vi "canDataSort.vi"() -> ()   [LabVIEW 2023] (continued)
 00000004    8        00\t00\tFF\tFF\tFF\tFF\tFF\tFF\r\n      2683  0CF102A7   00000004    8        30\t75\tE0\t2E\t80\tFF\tFF\tFD\r\n      2683  0CF101A7   00000004    8        68\t00\t97\tCC\t00\t16\t39\tA0\r\n      2682  1FFFFFFF   00000004    8        00\t20\tFF\tFF\tFF\tFF\tFF\tFF\r\n      2672  1FFFFFFF   00000004    8        00\t00\tFF\tFF\tFF\tFF\tFF\tFF\r\n      2663  0CF102A7   00000004    8        30\t75\tE0\t2E\t80\tFF\tFF\tFD\r\n      2663  0CF101A7   00000004    8        68\t00\t97\tCC\t00\t16\t39\t9F\r\n      2662  1FFFFFFF   00000004    8        00\t00\tFF\tFF\tFF\tFF\tFF\tFF\r\n      2652  1FFFFFFF   00000004    8        00\t00\tFF\tFF\tFF\tFF\tFF\tFF\r\n      2703  0CF101A7   00000004    8        68\t00\t97\tCC\t00\t16\t39\tA1\r\n      2702  1FFFFFFF   00000004    8        00\t00\tFF\tFF\tFF\tFF\tFF\tFF\r\n      2693  18F106A7   00000004    8        00\tF7\tFF\tFF\tFF\tFF\tFF\tA6\r\n      2692  1FFFFFFF   00000004    8        00\t00\tFF\tFF\tFF\tFF\tFF\tFF\r\n      2683  0CF102A7   00000004    8        30\t75\tE0\t2E\t80\tFF\tFF\tFD\r\n      2683  0CF101A7   00000004    8        68\t00\t97\tCC\t00\t16\t39\tA0\r\n      2682  1FFFFFFF   00000004    8        00\t20\tFF\tFF\tFF\tFF\tFF\tFF\r\n      2672  1FFFFFFF   00000004    8        00\t00\tFF\tFF\tFF\tFF\tFF\tFF\r\n      2663  0CF102A7   00000004    8        30\t75\tE0\t2E\t80\tFF\tFF\tFD\r\n      2663  0CF101A7   00000004    8        68\t00\t97\tCC\t00\t16\t39\t9F\r\n      2662  1FFFFFFF   00000004    8        00\t00\tFF\tFF\tFF\tFF\tFF\tFF\r\n      2703  0CF102A7   00000004    8        30\t75\tE0\t2E\t80\tFF\tFF\tFD\r\n      2703  0CF101A7   00000004    8        68\t00\t97\tCC\t00\t16\t39\tA1\r\n      2702  1FFFFFFF   00000004    8        00\t00\tFF\tFF\tFF\tFF\tFF\tFF\r\n      2693  18F106A7   00000004    8        00\tF7\tFF\tFF\tFF\tFF\tFF\tA6\r\n      2692  1FFFFFFF   00000004    8        00\t00\tFF\tFF\tFF\tFF\tFF\tFF\r\n      2683  0CF102A7   00000004    8        30\t75\tE0\t2E\t80\tFF\tFF\tFD\r\n      2683  0CF101A7   00000004    8        68\t00\t97\tCC\t00\t16\t39\tA0\r\n      2682  1FFFFFFF   00000004    8        00\t20\tFF\tFF\tFF\tFF\tFF\tFF\r\n      2672  1FFFFFFF   00000004    8        00\t00\tFF\tFF\tFF\tFF\tFF\tFF\r\n      2663  0CF102A7   00000004    8        30\t75\tE0\t2E\t80\tFF\tFF\tFD\r\n      2663  0CF101A7   00000004    8        68\t00\t97\tCC\t00\t16\t39\t9F\r\n      2712  1FFFFFFF   00000004    8        00\t00\tFF\tFF\tFF\tFF\tFF\tFF\r\n      2703  0CF102A7   00000004    8        30\t75\tE0\t2E\t80\tFF\tFF\tFD\r\n      2703  0CF101A7   00000004    8        68\t00\t97\tCC\t00\t16\t39\tA1\r\n      2702  1FFFFFFF   00000004    8        00\t00\tFF\tFF\tFF\tFF\tFF\tFF\r\n      2693  18F106A7   00000004    8        00\tF7\tFF\tFF\tFF\tFF\tFF\tA6\r\n      2692  1FFFFFFF   00000004    8        00\t00\tFF\tFF\tFF\tFF\tFF\tFF\r\n      2683  0CF102A7   00000004    8        30\t75\tE0\t2E\t80\tFF\tFF\tFD\r\n      2683  0CF101A7   00000004    8        68\t00\t97\tCC\t00\t16\t39\tA0\r\n      2682  1FFFFFFF   00000004    8        00\t20\tFF\tFF\tFF\tFF\tFF\tFF\r\n      2672  1FFFFFFF   00000004    8        00\t00\tFF\tFF\tFF\tFF\tFF\tFF\r\n      2663  0CF102A7   00000004    8        30\t75\tE0\t2E\t80\tFF\tFF\tFD\r\n      2722  1FFFFFFF   00000004    8        00\t00\tFF\tFF\tFF\tFF\tFF\tFF\r\n      2712  1FFFFFFF   00000004    8        00\t00\tFF\tFF\tFF\tFF\tFF\tFF\r\n      2703  0CF102A7   00000004    8        30\t75\tE0\t2E\t80\tFF\tFF\tFD\r\n      2703  0CF101A7   00000004    8        68\t00\t97\tCC\t00\t16\t39\tA1\r\n      2702  1FFFFFFF   00000004    8        00\t00\tFF\tFF\tFF\tFF\tFF\tFF\r\n      2693  18F106A7   00000004    8        00\tF7\tFF\tFF\tFF\tFF\tFF\tA6\r\n      2692  1FFFFFFF   00000004    8        00\t00\tFF\tFF\tFF\tFF\tFF\tFF\r\n      2683  0CF102A7   00000004    8        30\t75\tE0\t2E\t80\tFF\tFF\tFD\r\n      2683  0CF101A7   00000004    8        68\t00\t97\tCC\t00\t16\t39\tA0\r\n      2682  1FFFFFFF   00000004    8        00\t20\tFF\tFF\tFF\tFF\tFF\tFF\r\n      2672  1FFFFFFF   00000004    8        00\t00\tFF\tFF\tFF\tFF\tFF\tFF\r\n      2723  0CF101A7   00000004    8        68\t00\t97\tCC\t00\t16\t39\tA2\r\n      2722  1FFFFFFF   00000004    8        00\t00\tFF\tFF\tFF\tFF\tFF\tFF\r\n      2712  1FFFFFFF   00000004    8        00\t00\tFF\tFF\tFF\tFF\tFF\tFF\r\n      2703  0CF102A7   00000004    8        30\t75\tE0\t2E\t80\tFF\tFF\tFD\r\n      2703  0CF101A7   00000004    8        68\t00\t97\tCC\t00\t16\t39\tA1\r\n      2702  1FFFFFFF   00000004    8        00\t00\tFF\tFF\tFF\tFF\tFF\tFF\r\n      2693  18F106A7   00000004    8        00\tF7\tFF\tFF\tFF\tFF\tFF\tA6\r\n      2692  1FFFFFFF   00000004    8        00\t00\tFF\tFF\tFF\tFF\tFF\tFF\r\n      2683  0CF102A7   00000004    8        30\t75\tE0\t2E\t80\tFF\tFF\tFD\r\n      2683  0CF101A7   00000004    8        68\t00\t97\tCC\t00\t16\t39\tA0\r\n      2682  1FFFFFFF   00000004    8        00\t20\tFF\tFF\tFF\tFF\tFF\tFF\r\n      2723  0CF102A7   00000004    8        30\t75\tE0\t2E\t80\tFF\tFF\tFD\r\n      2723  0CF101A7   00000004    8        68\t00\t97\tCC\t00\t16\t39\tA2\r\n      2722  1FFFFFFF   00000004    8        00\t00\tFF\tFF\tFF\tFF\tFF\tFF\r\n      2712  1FFFFFFF   00000004    8        00\t00\tFF\tFF\tFF\tFF\tFF\tFF\r\n      2703  0CF102A7   00000004    8        30\t75\tE0\t2E\t80\tFF\tFF\tFD\r\n      2703  0CF101A7   00000004    8        68\t00\t97\tCC\t00\t16\t39\tA1\r\n      2702  1FFFFFFF   00000004    8        00\t00\tFF\tFF\tFF\tFF\tFF\tFF\r\n      2693  18F106A7   00000004    8        00\tF7\tFF\tFF\tFF\tFF\tFF\tA6\r\n      2692  1FFFFFFF   00000004    8        00\t00\tFF\tFF\tFF\tFF\tFF\tFF\r\n      2683  0CF102A7   00000004    8        30\t75\tE0\t2E\t80\tFF\tFF\tFD\r\n      2683  0CF101A7   00000004    8        68\t00\t97\tCC\t00\t16\t39\tA0\r\n      2732  1FFFFFFF   00000004    8        00\t00\tFF\tFF\tFF\tFF\tFF\tFF\r\n      2723  0CF102A7   00000004    8        30\t75\tE0\t2E\t80\tFF\tFF\tFD\r\n      2723  0CF101A7   00000004    8        68\t00\t97\tCC\t00\t16\t39\tA2\r\n      2722  1FFFFFFF   00000004    8        00\t00\tFF\tFF\tFF\tFF\tFF\tFF\r\n      2712  1FFFFFFF   00000004    8        00\t00\tFF\tFF\tFF\tFF\tFF\tFF\r\n      2703  0CF102A7   00000004    8        30\t75\tE0\t2E\t80\tFF\tFF\tFD\r\n      2703  0CF101A7   00000004    8        68\t00\t97\tCC\t00\t16\t39\tA1\r\n      2702  1FFFFFFF   00000004    8        00\t00\tFF\tFF\tFF\tFF\tFF\tFF\r\n      2693  18F106A7   00000004    8        00\tF7\tFF\tFF\tFF\tFF\tFF\tA6\r\n      2692  1FFFFFFF   00000004    8        00\t00\tFF\tFF\tFF\tFF\tFF\tFF\r\n      2683  0CF102A7   00000004    8        30\t75\tE0\t2E\t80\tFF\tFF\tFD\r\n      2741  18F11FF0   00000004    8        FF\t3F\t90\t68\t88\t1B\t10\t3C\r\n      2732  1FFFFFFF   00000004    8        00\t00\tFF\tFF\tFF\tFF\tFF\tFF\r\n      2723  0CF102A7   00000004    8        30\t75\tE0\t2E\t80\tFF\tFF\tFD\r\n      2723  0CF101A7   00000004    8        68\t00\t97\tCC\t00\t16\t39\tA2\r\n      2722  1FFFFFFF   00000004    8        00\t00\tFF\tFF\tFF\tFF\tFF\tFF\r\n      2712  1FFFFFFF   00000004    8        00\t00\tFF\tFF\tFF\tFF\tFF\tFF\r\n      2703  0CF102A7   00000004    8        30\t75\tE0\t2E\t80\tFF\tFF\tFD\r\n      2703  0CF101A7   00000004    8        68\t00\t97\tCC\t00\t16\t39\tA1\r\n      2702  1FFFFFFF   00000004    8        00\t00\tFF\tFF\tFF\tFF\tFF\tFF\r\n      2693  18F106A7   00000004    8        00\tF7\tFF\tFF\tFF\tFF\tFF\tA6\r\n      2692  1FFFFFFF   00000004    8        00\t00\tFF\tFF\tFF\tFF\tFF\tFF\r\n      2742  18F120F0   00000004    8        2B\t75\t60\tB1\tB0\t01\tFF\tFF\r\n      2741  18F11FF0   00000004    8        FF\t3F\t90\t68\t88\t1B\t10\t3C\r\n      2732  1FFFFFFF   00000004    8        00\t00\tFF\tFF\tFF\tFF\tFF\tFF\r\n      2723  0CF102A7   00000004    8        30\t75\tE0\t2E\t80\tFF\tFF\tFD\r\n      2723  0CF101A7   00000004    8        68\t00\t97\tCC\t00\t16\t39\tA2\r\n      2722  1FFFFFFF   00000004    8        00\t00\tFF\tFF\tFF\tFF\tFF\tFF\r\n      2712  1FFFFFFF   00000004    8        00\t00\tFF\tFF\tFF\tFF\tFF\tFF\r\n      2703  0CF102A7   00000004    8        30\t75\tE0\t2E\t80\tFF\tFF\tFD\r\n      2703  0CF101A7   00000004    8        68\t00\t97\tCC\t00\t16\t39\tA1\r\n      2702  1FFFFFFF   00000004    8        00\t00\tFF\tFF\tFF\tFF\tFF\tFF\r\n      2693  18F106A7   00000004    8        00\tF7\tFF\tFF\tFF\tFF\tFF\tA6\r\n      2743  0CF101A7   00000004    8        68\t00\t97\tCC\t00\t16\t39\tA3\r\n      2742  18F120F0   00000004    8        2B\t75\t60\tB1\tB0\t01\tFF\tFF\r\n      2741  18F11FF0   00000004    8        FF\t3F\t90\t68\t88\t1B\t10\t3C\r\n      2732  1FFFFFFF   00000004    8        00\t00\tFF\tFF\tFF\tFF\tFF\tFF\r\n      2723  0CF102A7   00000004    8        30\t75\tE0\t2E\t80\tFF\tFF\tFD\r\n      2723  0CF101A7   00000004    8        68\t00\t97\tCC\t00\t16\t39\tA2\r\n      2722  1FFFFFFF   00000004    8        00\t00\tFF\tFF\tFF\tFF\tFF\tFF\r\n      2712  1FFFFFFF   00000004    8        00\t00\tFF\tFF\tFF\tFF\tFF\tFF\r\n      2703  0CF102A7   00000004    8        30\t75\tE0\t2E\t80\tFF\tFF\tFD\r\n      2703  0CF101A7   00000004    8        68\t00\t97\tCC\t00\t16\t39\tA1\r\n      2702  1FFFFFFF   00000004    8        00\t00\tFF\tFF\tFF\tFF\tFF\tFF\r\n      2743  0C3C4D4A   00000004    8        BE\tFF\tFF\t7F\t18\tFF\tFF\t53\r\n      2743  0CF101A7   00000004    8        68\t00\t97\tCC\t00\t16\t39\tA3\r\n      2742  18F120F0   00000004    8        2B\t75\t60\tB1\tB0\t01\tFF\tFF\r\n      2741  18F11FF0   00000004    8        FF\t3F\t90\t68\t88\t1B\t10\t3C\r\n      2732  1FFFFFFF   00000004    8        00\t00\tFF\tFF\tFF\tFF\tFF\tFF\r\n      2723  0CF102A7   00000004    8        30\t75\tE0\t2E\t80\tFF\tFF\tFD\r\n      2723  0CF101A7   00000004    8        68\t00\t97\tCC\t00\t16\t39\tA2\r\n      2722  1FFFFFFF   00000004    8        00\t00\tFF\tFF\tFF\tFF\tFF\tFF\r\n      2712  1FFFFFFF   00000004    8        00\t00\tFF\tFF\tFF\tFF\tFF\tFF\r\n      2703  0CF102A7   00000004    8        30\t75\tE0\t2E\t80\tFF\tFF\tFD\r\n      2703  0CF101A7   00000004    8        68\t00\t97\tCC\t00\t16\t39\tA1\r\n      2744  0CF102A7   00000004    8        30\t75\tE0\t2E\t80\tFF\tFF\tFD\r\n      2743  0C3C4D4A   00000004    8        BE\tFF\tFF\t7F\t18\tFF\tFF\t53\r\n      2743  0CF101A7   00000004    8        68\t00\t97\tCC\t00\t16\t39\tA3\r\n      2742  18F120F0   00000004    8        2B\t75\t60\tB1\tB0\t01\tFF\tFF\r\n      2741  18F11FF0   00000004    8        FF\t3F\t90\t68\t88\t1B\t10\t3C\r\n      2732  1FFFFFFF   00000004    8        00\t00\tFF\tFF\tFF\tFF\tFF\tFF\r\n      2723  0CF102A7   00000004    8        30\t75\tE0\t2E\t80\tFF\tFF\tFD\r\n      2723  0CF101A7   00000004    8        68\t00\t97\tCC\t00\t16\t39\tA2\r\n      2722  1FFFFFFF   00000004    8        00\t00\tFF\tFF\tFF\tFF\tFF\tFF\r\n      2712  1FFFFFFF   00000004    8        00\t00\tFF\tFF\tFF\tFF\tFF\tFF\r\n      2703  0CF102A7   00000004    8        30\t75\tE0\t2E\t80\tFF\tFF\tFD\r\n      2744  0CF103A7   00000004    8        17\t1F\t08\t60\tB1\t1F\t08\t53\r\n      2744  0CF102A7   00000004    8        30\t75\tE0\t2E\t80\tFF\tFF\tFD\r\n      2743  0C3C4D4A   00000004    8        BE\tFF\tFF\t7F\t18\tFF\tFF\t53\r\n      2743  0CF101A7   00000004    8        68\t00\t97\tCC\t00\t16\t39\tA3\r\n      2742  18F120F0   00000004    8        2B\t75\t60\tB1\tB0\t01\tFF\tFF\r\n      2741  18F11FF0   00000004    8        FF\t3F\t90\t68\t88\t1B\t10\t3C\r\n      2732  1FFFFFFF   00000004    8        00\t00\tFF\tFF\tFF\tFF\tFF\tFF\r\n      2723  0CF102A7   00000004    8        30\t75\tE0\t2E\t80\tFF\tFF\tFD\r\n      2723  0CF101A7   00000004    8        68\t00\t97\tCC\t00\t16\t39\tA2\r\n      2722  1FFFFFFF   00000004    8        00\t00\tFF\tFF\tFF\tFF\tFF\tFF\r\n      2712  1FFFFFFF   00000004    8        00\t00\tFF\tFF\tFF\tFF\tFF\tFF\r\n      2745  0CF104A7   00000004    8        F0\t60\t22\tFC\tFF\tFF\tFF\t53\r\n      2744  0CF103A7   00000004    8        17\t1F\t08\t60\tB1\t1F\t08\t53\r\n      2744  0CF102A7   00000004    8        30\t75\tE0\t2E\t80\tFF\tFF\tFD\r\n      2743  0C3C4D4A   00000004    8        BE\tFF\tFF\t7F\t18\tFF\tFF\t53\r\n      2743  0CF101A7   00000004    8        68\t00\t97\tCC\t00\t16\t39\tA3\r\n      2742  18F120F0   00000004    8        2B\t75\t60\tB1\tB0\t01\tFF\tFF\r\n      2741  18F11FF0   00000004    8        FF\t3F\t90\t68\t88\t1B\t10\t3C\r\n      2732  1FFFFFFF   00000004    8        00\t00\tFF\tFF\tFF\tFF\tFF\tFF\r\n      2723  0CF102A7   00000004    8        30\t75\tE0\t2E\t80\tFF\tFF\tFD\r\n      2723  0CF101A7   00000004    8        68\t00\t97\tCC\t00\t16\t39\tA2\r\n      2722  1FFFFFFF   00000004    8        00\t00\tFF\tFF\tFF\tFF\tFF\tFF\r\n      2745  18F106A7   00000004    8        00\tF7\tFF\tFF\tFF\tFF\tFF\tA7\r\n      2745  0CF104A7   00000004    8        F0\t60\t22\tFC\tFF\tFF\tFF\t53\r\n      2744  0CF103A7   00000004    8        17\t1F\t08\t60\tB1\t1F\t08\t53\r\n      2744  0CF102A7   00000004    8        30\t75\tE0\t2E\t80\tFF\tFF\tFD\r\n      2743  0C3C4D4A   00000004    8        BE\tFF\tFF\t7F\t18\tFF\tFF\t53\r\n      2743  0CF101A7   00000004    8        68\t00\t97\tCC\t00\t16\t39\tA3\r\n      2742  18F120F0   00000004    8        2B\t75\t60\tB1\tB0\t01\tFF\tFF\r\n      2741  18F11FF0   00000004    8        FF\t3F\t90\t68\t88\t1B\t10\t3C\r\n      2732  1FFFFFFF   00000004    8        00\t00\tFF\tFF\tFF\tFF\tFF\tFF\r\n      2723  0CF102A7   00000004    8        30\t75\tE0\t2E\t80\tFF\tFF\tFD\r\n      2723  0CF101A7   00000004    8        68\t00\t97\tCC\t00\t16\t39\tA2\r\n      2746  18F121F0   00000004    8        09\t19\t00\t00\tFF\tFF\tB0\t01\r\n      2745  18F106A7   00000004    8        00\tF7\tFF\tFF\tFF\tFF\tFF\tA7\r\n      2745  0CF104A7   00000004    8        F0\t60\t22\tFC\tFF\tFF\tFF\t53\r\n      2744  0CF103A7   00000004    8        17\t1F\t08\t60\tB1\t1F\t08\t53\r\n      2744  0CF102A7   00000004    8        30\t75\tE0\t2E\t80\tFF\tFF\tFD\r\n      2743  0C3C4D4A   00000004    8        BE\tFF\tFF\t7F\t18\tFF\tFF\t53\r\n      2743  0CF101A7   00000004    8        68\t00\t97\tCC\t00\t16\t39\tA3\r\n      2742  18F120F0   00000004    8        2B\t75\t60\tB1\tB0\t01\tFF\tFF\r\n      2741  18F11FF0   00000004    8        FF\t3F\t90\t68\t88\t1B\t10\t3C\r\n      2732  1FFFFFFF   00000004    8        00\t00\tFF\tFF\tFF\tFF\tFF\tFF\r\n      2723  0CF102A7   00000004    8        30\t75\tE0\t2E\t80\tFF\tFF\tFD\r\n      2747  1FFFFFFF   00000004    8        00\t00\tFF\tFF\tFF\tFF\tFF\tFF\r\n      2746  18F121F0   00000004    8        09\t19\t00\t00\tFF\tFF\tB0\t01\r\n      2745  18F106A7   00000004    8        00\tF7\tFF\tFF\tFF\tFF\tFF\tA7\r\n      2745  0CF104A7   00000004    8        F0\t60\t22\tFC\tFF\tFF\tFF\t53\r\n      2744  0CF103A7   00000004    8        17\t1F\t08\t60\tB1\t1F\t08\t53\r\n      2744  0CF102A7   00000004    8        30\t75\tE0\t2E\t80\tFF\tFF\tFD\r\n      2743  0C3C4D4A   00000004    8        BE\tFF\tFF\t7F\t18\tFF\tFF\t53\r\n      2743  0CF101A7   00000004    8        68\t00\t97\tCC\t00\t16\t39\tA3\r\n      2742  18F120F0   00000004    8        2B\t75\t60\tB1\tB0\t01\tFF\tFF\r\n      2741  18F11FF0   00000004    8        FF\t3F\t90\t68\t88\t1B\t10\t3C\r\n      2732  1FFFFFFF   00000004    8        00\t00\tFF\tFF\tFF\tFF\tFF\tFF\r\n      2752  1FFFFFFF   00000004    8        00\t00\tFF\tFF\tFF\tFF\tFF\tFF\r\n      2747  1FFFFFFF   00000004    8        00\t00\tFF\tFF\tFF\tFF\tFF\tFF\r\n      2746  18F121F0   00000004    8        09\t19\t00\t00\tFF\tFF\tB0\t01\r\n      2745  18F106A7   00000004    8        00\tF7\tFF\tFF\tFF\tFF\tFF\tA7\r\n      2745  0CF104A7   00000004    8        F0\t60\t22\tFC\tFF\tFF\tFF\t53\r\n      2744  0CF103A7   00000004    8        17\t1F\t08\t60\tB1\t1F\t08\t53\r\n      2744  0CF102A7   00000004    8        30\t75\tE0\t2E\t80\tFF\tFF\tFD\r\n      2743  0C3C4D4A   00000004    8        BE\tFF\tFF\t7F\t18\tFF\tFF\t53\r\n      2743  0CF101A7   00000004    8        68\t00\t97\tCC\t00\t16\t39\tA3\r\n      2742  18F120F0   00000004    8        2B\t75\t60\tB1\tB0\t01\tFF\tFF\r\n      2741  18F11FF0   00000004    8        FF\t3F\t90\t68\t88\t1B\t10\t3C\r\n      2762  1FFFFFFF   00000004    8        00\t00\tFF\tFF\tFF\tFF\tFF\tFF\r\n      2752  1FFFFFFF   00000004    8        00\t00\tFF\tFF\tFF\tFF\tFF\tFF\r\n      2747  1FFFFFFF   00000004    8        00\t00\tFF\tFF\tFF\tFF\tFF\tFF\r\n      2746  18F121F0   00000004    8        09\t19\t00\t00\tFF\tFF\tB0\t01\r\n      2745  18F106A7   00000004    8        00\tF7\tFF\tFF\tFF\tFF\tFF\tA7\r\n      2745  0CF104A7   00000004    8        F0\t60\t22\tFC\tFF\tFF\tFF\t53\r\n      2744  0CF103A7   00000004    8        17\t1F\t08\t60\tB1\t1F\t08\t53\r\n      2744  0CF102A7   00000004    8        30\t75\tE0\t2E\t80\tFF\tFF\tFD\r\n      2743  0C3C4D4A   00000004    8        BE\tFF\tFF\t7F\t18\tFF\tFF\t53\r\n      2743  0CF101A7   00000004    8        68\t00\t97\tCC\t00\t16\t39\tA3\r\n      2742  18F120F0   00000004    8        2B\t75\t60\tB1\tB0\t01\tFF\tFF\r\n      2763  0CF101A7   00000004    8        68\t00\t97\tCC\t00\t16\t39\tA4\r\n      2762  1FFFFFFF   00000004    8        00\t00\tFF\tFF\tFF\tFF\tFF\tFF\r\n      2752  1FFFFFFF   00000004    8        00\t00\tFF\tFF\tFF\tFF\tFF\tFF\r\n      2747  1FFFFFFF   00000004    8        00\t00\tFF\tFF\tFF\tFF\tFF\tFF\r\n      2746  18F121F0   00000004    8        09\t19\t00\t00\tFF\tFF\tB0\t01\r\n      2745  18F106A7   00000004    8        00\tF7\tFF\tFF\tFF\tFF\tFF\tA7\r\n      2745  0CF104A7   00000004    8        F0\t60\t22\tFC\tFF\tFF\tFF\t53\r\n      2744  0CF103A7   00000004    8        17\t1F\t08\t60\tB1\t1F\t08\t53\r\n      2744  0CF102A7   00000004    8        30\t75\tE0\t2E\t80\tFF\tFF\tFD\r\n      2743  0C3C4D4A   00000004    8        BE\tFF\tFF\t7F\t18\tFF\tFF\t53\r\n      2743  0CF101A7   00000004    8        68\t00\t97\tCC\t00\t16\t39\tA3\r\n      2763  0CF102A7   00000004    8        30\t75\tE0\t2E\t80\tFF\tFF\tFD\r\n      2763  0CF101A7   00000004    8        68\t00\t97\tCC\t00\t16\t39\tA4\r\n      2762  1FFFFFFF   00000004    8        00\t00\tFF\tFF\tFF\tFF\tFF\tFF\r\n      2752  1FFFFFFF   00000004    8        00\t00\tFF\tFF\tFF\tFF\tFF\tFF\r\n      2747  1FFFFFFF   00000004    8        00\t00\tFF\tFF\tFF\tFF\tFF\tFF\r\n      2746  18F121F0   00000004    8        09\t19\t00\t00\tFF\tFF\tB0\t01\r\n      2745  18F106A7   00000004    8        00\tF7\tFF\tFF\tFF\tFF\tFF\tA7\r\n      2745  0CF104A7   00000004    8        F0\t60\t22\tFC\tFF\tFF\tFF\t53\r\n      2744  0CF103A7   00000004    8        17\t1F\t08\t60\tB1\t1F\t08\t53\r\n      2744  0CF102A7   00000004    8        30\t75\tE0\t2E\t80\tFF\tFF\tFD\r\n      2743  0C3C4D4A   00000004    8        BE\tFF\tFF\t7F\t18\tFF\tFF\t53\r\n      2772  1FFFFFFF   00000004    8        00\t00\tFF\tFF\tFF\tFF\tFF\tFF\r\n      2763  0CF102A7   00000004    8        30\t75\tE0\t2E\t80\tFF\tFF\tFD\r\n      2763  0CF101A7   00000004    8        68\t00\t97\tCC\t00\t16\t39\tA4\r\n      2762  1FFFFFFF   00000004    8        00\t00\tFF\tFF\tFF\tFF\tFF\tFF\r\n      2752  1FFFFFFF   00000004    8        00\t00\tFF\tFF\tFF\tFF\tFF\tFF\r\n      2747  1FFFFFFF   00000004    8        00\t00\tFF\tFF\tFF\tFF\tFF\tFF\r\n      2746  18F121F0   00000004    8        09\t19\t00\t00\tFF\tFF\tB0\t01\r\n      2745  18F106A7   00000004    8        00\tF7\tFF\tFF\tFF\tFF\tFF\tA7\r\n      2745  0CF104A7   00000004    8        F0\t60\t22\tFC\tFF\tFF\tFF\t53\r\n      2744  0CF103A7   00000004    8        17\t1F\t08\t60\tB1\t1F\t08\t53\r\n      2744  0CF102A7   00000004    8        30\t75\tE0\t2E\t80\tFF\tFF\tFD\r\n      2782  1FFFFFFF   00000004    8        00\t00\tFF\tFF\tFF\tFF\tFF\tFF\r\n      2772  1FFFFFFF   00000004    8        00\t00\tFF\tFF\tFF\tFF\tFF\tFF\r\n      2763  0CF102A7   00000004    8        30\t75\tE0\t2E\t80\tFF\tFF\tFD\r\n      2763  0CF101A7   00000004    8        68\t00\t97\tCC\t00\t16\t39\tA4\r\n      2762  1FFFFFFF   00000004    8        00\t00\tFF\tFF\tFF\tFF\tFF\tFF\r\n      2752  1FFFFFFF   00000004    8        00\t00\tFF\tFF\tFF\tFF\tFF\tFF\r\n      2747  1FFFFFFF   00000004    8        00\t00\tFF\tFF\tFF\tFF\tFF\tFF\r\n      2746  18F121F0   00000004    8        09\t19\t00\t00\tFF\tFF\tB0\t01\r\n      2745  18F106A7   00000004    8        00\tF7\tFF\tFF\tFF\tFF\tFF\tA7\r\n      2745  0CF104A7   00000004    8        F0\t60\t22\tFC\tFF\tFF\tFF\t53\r\n      2744  0CF103A7   00000004    8        17\t1F\t08\t60\tB1\t1F\t08\t53\r\n      2783  0CF101A7   00000004    8        68\t00\t97\tCC\t00\t16\t39\tA5\r\n      2782  1FFFFFFF   00000004    8        00\t00\tFF\tFF\tFF\tFF\tFF\tFF\r\n      2772  1FFFFFFF   00000004    8        00\t00\tFF\tFF\tFF\tFF\tFF\tFF\r\n      2763  0CF102A7   00000004    8        30\t75\tE0\t2E\t80\tFF\tFF\tFD\r\n      2763  0CF101A7   00000004    8        68\t00\t97\tCC\t00\t16\t39\tA4\r\n      2762  1FFFFFFF   00000004    8        00\t00\tFF\tFF\tFF\tFF\tFF\tFF\r\n      2752  1FFFFFFF   00000004    8        00\t00\tFF\tFF\tFF\tFF\tFF\tFF\r\n      2747  1FFFFFFF   00000004    8        00\t00\tFF\tFF\tFF\tFF\tFF\tFF\r\n      2746  18F121F0   00000004    8        09\t19\t00\t00\tFF\tFF\tB0\t01\r\n      2745  18F106A7   00000004    8        00\tF7\tFF\tFF\tFF\tFF\tFF\tA7\r\n      2745  0CF104A7   00000004    8        F0\t60\t22\tFC\tFF\tFF\tFF\t53\r\n      2783  0CF102A7   00000004    8        30\t75\tE0\t2E\t80\tFF\tFF\tFD\r\n      2783  0CF101A7   00000004    8        68\t00\t97\tCC\t00\t16\t39\tA5\r\n      2782  1FFFFFFF   00000004    8        00\t00\tFF\tFF\tFF\tFF\tFF\tFF\r\n      2772  1FFFFFFF   00000004    8        00\t00\tFF\tFF\tFF\tFF\tFF\tFF\r\n      2763  0CF102A7   00000004    8        30\t75\tE0\t2E\t80\tFF\tFF\tFD\r\n      2763  0CF101A7   00000004    8        68\t00\t97\tCC\t00\t16\t39\tA4\r\n      2762  1FFFFFFF   00000004    8        00\t00\tFF\tFF\tFF\tFF\tFF\tFF\r\n      2752  1FFFFFFF   00000004    8        00\t00\tFF\tFF\tFF\tFF\tFF\tFF\r\n      2747  1FFFFFFF   00000004    8        00\t00\tFF\tFF\tFF\tFF\tFF\tFF\r\n      2746  18F121F0   00000004    8        09\t19\t00\t00\tFF\tFF\tB0\t01\r\n      2745  18F106A7   00000004    8        00\tF7\tFF\tFF\tFF\tFF\tFF\tA7\r\n      2792  1FFFFFFF   00000004    8        00\t00\tFF\tFF\tFF\tFF\tFF\tFF\r\n      2783  0CF102A7   00000004    8        30\t75\tE0\t2E\t80\tFF\tFF\tFD\r\n      2783  0CF101A7   00000004    8        68\t00\t97\tCC\t00\t16\t39\tA5\r\n      2782  1FFFFFFF   00000004    8        00\t00\tFF\tFF\tFF\tFF\tFF\tFF\r\n      2772  1FFFFFFF   00000004    8        00\t00\tFF\tFF\tFF\tFF\tFF\tFF\r\n      2763  0CF102A7   00000004    8        30\t75\tE0\t2E\t80\tFF\tFF\tFD\r\n      2763  0CF101A7   00000004    8        68\t00\t97\tCC\t00\t16\t39\tA4\r\n      2762  1FFFFFFF   00000004    8        00\t00\tFF\tFF\tFF\tFF\tFF\tFF\r\n      2752  1FFFFFFF   00000004    8        00\t00\tFF\tFF\tFF\tFF\tFF\tFF\r\n      2747  1FFFFFFF   00000004    8        00\t00\tFF\tFF\tFF\tFF\tFF\tFF\r\n      2746  18F121F0   00000004    8        09\t19\t00\t00\tFF\tFF\tB0\t01\r\n      2793  18F106A7   00000004    8        00\tF7\tFF\tFF\tFF\tFF\tFF\tA8\r\n      2792  1FFFFFFF   00000004    8        00\t00\tFF\tFF\tFF\tFF\tFF\tFF\r\n      2783  0CF102A7   00000004    8        30\t75\tE0\t2E\t80\tFF\tFF\tFD\r\n      2783  0CF101A7   00000004    8        68\t00\t97\tCC\t00\t16\t39\tA5\r\n      2782  1FFFFFFF   00000004    8        00\t00\tFF\tFF\tFF\tFF\tFF\tFF\r\n      2772  1FFFFFFF   00000004    8        00\t00\tFF\tFF\tFF\tFF\tFF\tFF\r\n      2763  0CF102A7   00000004    8        30\t75\tE0\t2E\t80\tFF\tFF\tFD\r\n      2763  0CF101A7   00000004    8        68\t00\t97\tCC\t00\t16\t39\tA4\r\n      2762  1FFFFFFF   00000004    8        00\t00\tFF\tFF\tFF\tFF\tFF\tFF\r\n      2752  1FFFFFFF   00000004    8        00\t00\tFF\tFF\tFF\tFF\tFF\tFF\r\n      2747  1FFFFFFF   00000004    8        00\t00\tFF\tFF\tFF\tFF\tFF\tFF\r\n      2802  1FFFFFFF   00000004    8        00\t00\tFF\tFF\tFF\tFF\tFF\tFF\r\n      2793  18F106A7   00000004    8        00\tF7\tFF\tFF\tFF\tFF\tFF\tA8\r\n      2792  1FFFFFFF   00000004    8        00\t00\tFF\tFF\tFF\tFF\tFF\tFF\r\n      2783  0CF102A7   00000004    8        30\t75\tE0\t2E\t80\tFF\tFF\tFD\r\n      2783  0CF101A7   00000004    8        68\t00\t97\tCC\t00\t16\t39\tA5\r\n      2782  1FFFFFFF   00000004    8        00\t00\tFF\tFF\tFF\tFF\tFF\tFF\r\n      2772  1FFFFFFF   00000004    8        00\t00\tFF\tFF\tFF\tFF\tFF\tFF\r\n      2763  0CF102A7   00000004    8        30\t75\tE0\t2E\t80\tFF\tFF\tFD\r\n      2763  0CF101A7   00000004    8        68\t00\t97\tCC\t00\t16\t39\tA4\r\n      2762  1FFFFFFF   00000004    8        00\t00\tFF\tFF\tFF\tFF\tFF\tFF\r\n      2752  1FFFFFFF   00000004    8        00\t00\tFF\tFF\tFF\tFF\tFF\tFF\r\n      2803  0CF101A7   00000004    8        68\t00\t97\tCC\t00\t16\t39\tA6\r\n      2802  1FFFFFFF   00000004    8        00\t00\tFF\tFF\tFF\tFF\tFF\tFF\r\n      2793  18F106A7   00000004    8        00\tF7\tFF\tFF\tFF\tFF\tFF\tA8\r\n      2792  1FFFFFFF   00000004    8        00\t00\tFF\tFF\tFF\tFF\tFF\tFF\r\n      2783  0CF102A7   00000004    8        30\t75\tE0\t2E\t80\tFF\tFF\tFD\r\n      2783  0CF101A7   00000004    8        68\t00\t97\tCC\t00\t16\t39\tA5\r\n      2782  1FFFFFFF   00000004    8        00\t00\tFF\tFF\tFF\tFF\tFF\tFF\r\n      2772  1FFFFFFF   00000004    8        00\t00\tFF\tFF\tFF\tFF\tFF\tFF\r\n      2763  0CF102A7   00000004    8        30\t75\tE0\t2E\t80\tFF\tFF\tFD\r\n      2763  0CF101A7   00000004    8        68\t00\t97\tCC\t00\t16\t39\tA4\r\n      2762  1FFFFFFF   00000004    8        00\t00\tFF\tFF\tFF\tFF\tFF\tFF\r\n      2803  0CF102A7   00000004    8        30\t75\tE0\t2E\t80\tFF\tFF\tFD\r\n      2803  0CF101A7   00000004    8        68\t00\t97\tCC\t00\t16\t39\tA6\r\n      2802  1FFFFFFF   00000004    8        00\t00\tFF\tFF\tFF\tFF\tFF\tFF\r\n      2793  18F106A7   00000004    8        00\tF7\tFF\tFF\tFF\tFF\tFF\tA8\r\n      2792  1FFFFFFF   00000004    8        00\t00\tFF\tFF\tFF\tFF\tFF\tFF\r\n      2783  0CF102A7   00000004    8        30\t75\tE0\t2E\t80\tFF\tFF\tFD\r\n      2783  0CF101A7   00000004    8        68\t00\t97\tCC\t00\t16\t39\tA5\r\n      2782  1FFFFFFF   00000004    8        00\t00\tFF\tFF\tFF\tFF\tFF\tFF\r\n      2772  1FFFFFFF   00000004    8        00\t00\tFF\tFF\tFF\tFF\tFF\tFF\r\n      2763  0CF102A7   00000004    8        30\t75\tE0\t2E\t80\tFF\tFF\tFD\r\n      2763  0CF101A7   00000004    8        68\t00\t97\tCC\t00\t16\t39\tA4\r\n      2812  1FFFFFFF   00000004    8        00\t00\tFF\tFF\tFF\tFF\tFF\tFF\r\n      2803  0CF102A7   00000004    8        30\t75\tE0\t2E\t80\tFF\tFF\tFD\r\n      2803  0CF101A7   00000004    8        68\t00\t97\tCC\t00\t16\t39\tA6\r\n      2802  1FFFFFFF   00000004    8        00\t00\tFF\tFF\tFF\tFF\tFF\tFF\r\n      2793  18F106A7   00000004    8        00\tF7\tFF\tFF\tFF\tFF\tFF\tA8\r\n      2792  1FFFFFFF   00000004    8        00\t00\tFF\tFF\tFF\tFF\tFF\tFF\r\n      2783  0CF102A7   00000004    8        30\t75\tE0\t2E\t80\tFF\tFF\tFD\r\n      2783  0CF101A7   00000004    8        68\t00\t97\tCC\t00\t16\t39\tA5\r\n      2782  1FFFFFFF   00000004    8        00\t00\tFF\tFF\tFF\tFF\tFF\tFF\r\n      2772  1FFFFFFF   00000004    8        00\t00\tFF\tFF\tFF\tFF\tFF\tFF\r\n      2763  0CF102A7   00000004    8        30\t75\tE0\t2E\t80\tFF\tFF\tFD\r\n      2822  1FFFFFFF   00000004    8        00\t00\tFF\tFF\tFF\tFF\tFF\tFF\r\n      2812  1FFFFFFF   00000004    8        00\t00\tFF\tFF\tFF\tFF\tFF\tFF\r\n      2803  0CF102A7   00000004    8        30\t75\tE0\t2E\t80\tFF\tFF\tFD\r\n      2803  0CF101A7   00000004    8        68\t00\t97\tCC\t00\t16\t39\tA6\r\n      2802  1FFFFFFF   00000004    8        00\t00\tFF\tFF\tFF\tFF\tFF\tFF\r\n      2793  18F106A7   00000004    8        00\tF7\tFF\tFF\tFF\tFF\tFF\tA8\r\n      2792  1FFFFFFF   00000004    8        00\t00\tFF\tFF\tFF\tFF\tFF\tFF\r\n      2783  0CF102A7   00000004    8        30\t75\tE0\t2E\t80\tFF\tFF\tFD\r\n      2783  0CF101A7   00000004    8        68\t00\t97\tCC\t00\t16\t39\tA5\r\n      2782  1FFFFFFF   00000004    8        00\t00\tFF\tFF\tFF\tFF\tFF\tFF\r\n      2772  1FFFFFFF   00000004    8        00\t00\tFF\tFF\tFF\tFF\tFF\tFF\r\n      2823  0CF101A7   00000004    8        68\t00\t97\tCC\t00\t16\t39\tA7\r\n      2822  1FFFFFFF   00000004    8        00\t00\tFF\tFF\tFF\tFF\tFF\tFF\r\n      2812  1FFFFFFF   00000004    8        00\t00\tFF\tFF\tFF\tFF\tFF\tFF\r\n      2803  0CF102A7   00000004    8        30\t75\tE0\t2E\t80\tFF\tFF\tFD\r\n      2803  0CF101A7   00000004    8        68\t00\t97\tCC\t00\t16\t39\tA6\r\n      2802  1FFFFFFF   00000004    8        00\t00\tFF\tFF\tFF\tFF\tFF\tFF\r\n      2793  18F106A7   00000004    8        00\tF7\tFF\tFF\tFF\tFF\tFF\tA8\r\n      2792  1FFFFFFF   00000004    8        00\t00\tFF\tFF\tFF\tFF\tFF\tFF\r\n      2783  0CF102A7   00000004    8        30\t75\tE0\t2E\t80\tFF\tFF\tFD\r\n      2783  0CF101A7   00000004    8        68\t00\t97\tCC\t00\t16\t39\tA5\r\n      2782  1FFFFFFF   00000004    8        00\t00\tFF\tFF\tFF\tFF\tFF\tFF\r\n      2823  0CF102A7   00000004    8        30\t75\tE0\t2E\t80\tFF\tFF\tFD\r\n      2823  0CF101A7   00000004    8        68\t00\t97\tCC\t00\t16\t39\tA7\r\n      2822  1FFFFFFF   00000004    8        00\t00\tFF\tFF\tFF\tFF\tFF\tFF\r\n      2812  1FFFFFFF   00000004    8        00\t00\tFF\tFF\tFF\tFF\tFF\tFF\r\n      2803  0CF102A7   00000004    8        30\t75\tE0\t2E\t80\tFF\tFF\tFD\r\n      2803  0CF101A7   00000004    8        68\t00\t97\tCC\t00\t16\t39\tA6\r\n      2802  1FFFFFFF   00000004    8        00\t00\tFF\tFF\tFF\tFF\tFF\tFF\r\n      2793  18F106A7   00000004    8        00\tF7\tFF\tFF\tFF\tFF\tFF\tA8\r\n      2792  1FFFFFFF   00000004    8        00\t00\tFF\tFF\tFF\tFF\tFF\tFF\r\n      2783  0CF102A7   00000004    8        30\t75\tE0\t2E\t80\tFF\tFF\tFD\r\n      2783  0CF101A7   00000004    8        68\t00\t97\tCC\t00\t16\t39\tA5\r\n      2832  1FFFFFFF   00000004    8        00\t00\tFF\tFF\tFF\tFF\tFF\tFF\r\n      2823  0CF102A7   00000004    8        30\t75\tE0\t2E\t80\tFF\tFF\tFD\r\n      2823  0CF101A7   00000004    8        68\t00\t97\tCC\t00\t16\t39\tA7\r\n      2822  1FFFFFFF   00000004    8        00\t00\tFF\tFF\tFF\tFF\tFF\tFF\r\n      2812  1FFFFFFF   00000004    8        00\t00\tFF\tFF\tFF\tFF\tFF\tFF\r\n      2803  0CF102A7   00000004    8        30\t75\tE0\t2E\t80\tFF\tFF\tFD\r\n      2803  0CF101A7   00000004    8        68\t00\t97\tCC\t00\t16\t39\tA6\r\n      2802  1FFFFFFF   00000004    8        00\t00\tFF\tFF\tFF\tFF\tFF\tFF\r\n      2793  18F106A7   00000004    8        00\tF7\tFF\tFF\tFF\tFF\tFF\tA8\r\n      2792  1FFFFFFF   00000004    8        00\t00\tFF\tFF\tFF\tFF\tFF\tFF\r\n      2783  0CF102A7   00000004    8        30\t75\tE0\t2E\t80\tFF\tFF\tFD\r\n      2841  18F11FF0   00000004    8        FF\t3F\t90\t68\t88\t1B\t10\t4C\r\n      2832  1FFFFFFF   00000004    8        00\t00\tFF\tFF\tFF\tFF\tFF\tFF\r\n      2823  0CF102A7   00000004    8        30\t75\tE0\t2E\t80\tFF\tFF\tFD\r\n      2823  0CF101A7   00000004    8        68\t00\t97\tCC\t00\t16\t39\tA7\r\n      2822  1FFFFFFF   00000004    8        00\t00\tFF\tFF\tFF\tFF\tFF\tFF\r\n      2812  1FFFFFFF   00000004    8        00\t00\tFF\tFF\tFF\tFF\tFF\tFF\r\n      2803  0CF102A7   00000004    8        30\t75\tE0\t2E\t80\tFF\tFF\tFD\r\n      2803  0CF101A7   00000004    8        68\t00\t97\tCC\t00\t16\t39\tA6\r\n      2802  1FFFFFFF   00000004    8        00\t00\tFF\tFF\tFF\tFF\tFF\tFF\r\n      2793  18F106A7   00000004    8        00\tF7\tFF\tFF\tFF\tFF\tFF\tA8\r\n      2792  1FFFFFFF   00000004    8        00\t00\tFF\tFF\tFF\tFF\tFF\tFF\r\n      2842  18F120F0   00000004    8        2B\t75\t60\tB1\tB0\t01\tFF\tFF\r\n      2841  18F11FF0   00000004    8        FF\t3F\t90\t68\t88\t1B\t10\t4C\r\n      2832  1FFFFFFF   00000004    8        00\t00\tFF\tFF\tFF\tFF\tFF\tFF\r\n      2823  0CF102A7   00000004    8        30\t75\tE0\t2E\t80\tFF\tFF\tFD\r\n      2823  0CF101A7   00000004    8        68\t00\t97\tCC\t00\t16\t39\tA7\r\n      2822  1FFFFFFF   00000004    8        00\t00\tFF\tFF\tFF\tFF\tFF\tFF\r\n      2812  1FFFFFFF   00000004    8        00\t00\tFF\tFF\tFF\tFF\tFF\tFF\r\n      2803  0CF102A7   00000004    8        30\t75\tE0\t2E\t80\tFF\tFF\tFD\r\n      2803  0CF101A7   00000004    8        68\t00\t97\tCC\t00\t16\t39\tA6\r\n      2802  1FFFFFFF   00000004    8        00\t00\tFF\tFF\tFF\tFF\tFF\tFF\r\n      2793  18F106A7   00000004    8        00\tF7\tFF\tFF\tFF\tFF\tFF\tA8\r\n      2843  0CF101A7   00000004    8        68\t00\t97\tCC\t00\t16\t39\tA8\r\n      2842  18F120F0   00000004    8        2B\t75\t60\tB1\tB0\t01\tFF\tFF\r\n      2841  18F11FF0   00000004    8        FF\t3F\t90\t68\t88\t1B\t10\t4C\r\n      2832  1FFFFFFF   00000004    8        00\t00\tFF\tFF\tFF\tFF\tFF\tFF\r\n      2823  0CF102A7   00000004    8        30\t75\tE0\t2E\t80\tFF\tFF\tFD\r\n      2823  0CF101A7   00000004    8        68\t00\t97\tCC\t00\t16\t39\tA7\r\n      2822  1FFFFFFF   00000004    8        00\t00\tFF\tFF\tFF\tFF\tFF\tFF\r\n      2812  1FFFFFFF   00000004    8        00\t00\tFF\tFF\tFF\tFF\tFF\tFF\r\n      2803  0CF102A7   00000004    8        30\t75\tE0\t2E\t80\tFF\tFF\tFD\r\n      2803  0CF101A7   00000004    8        68\t00\t97\tCC\t00\t16\t39\tA6\r\n      2802  1FFFFFFF   00000004    8        00\t00\tFF\tFF\tFF\tFF\tFF\tFF\r\n      2843  0C3C4D4A   00000004    8        BE\tFF\tFF\t7F\t18\tFF\tFF\t54\r\n      2843  0CF101A7   00000004    8        68\t00\t97\tCC\t00\t16\t39\tA8\r\n      2842  18F120F0   00000004    8        2B\t75\t60\tB1\tB0\t01\tFF\tFF\r\n      2841  18F11FF0   00000004    8        FF\t3F\t90\t68\t88\t1B\t10\t4C\r\n      2832  1FFFFFFF   00000004    8        00\t00\tFF\tFF\tFF\tFF\tFF\tFF\r\n      2823  0CF102A7   00000004    8        30\t75\tE0\t2E\t80\tFF\tFF\tFD\r\n      2823  0CF101A7   00000004    8        68\t00\t97\tCC\t00\t16\t39\tA7\r\n      2822  1FFFFFFF   00000004    8        00\t00\tFF\tFF\tFF\tFF\tFF\tFF\r\n      2812  1FFFFFFF   00000004    8        00\t00\tFF\tFF\tFF\tFF\tFF\tFF\r\n      2803  0CF102A7   00000004    8        30\t75\tE0\t2E\t80\tFF\tFF\tFD\r\n      2803  0CF101A7   00000004    8        68\t00\t97\tCC\t00\t16\t39\tA6\r\n      2844  0CF102A7   00000004    8        30\t75\tE0\t2E\t80\tFF\tFF\tFD\r\n      2843  0C3C4D4A   00000004    8        BE\tFF\tFF\t7F\t18\tFF\tFF\t54\r\n      2843  0CF101A7   00000004    8        68\t00\t97\tCC\t00\t16\t39\tA8\r\n      2842  18F120F0   00000004    8        2B\t75\t60\tB1\tB0\t01\tFF\tFF\r\n      2841  18F11FF0   00000004    8        FF\t3F\t90\t68\t88\t1B\t10\t4C\r\n      2832  1FFFFFFF   00000004    8        00\t00\tFF\tFF\tFF\tFF\tFF\tFF\r\n      2823  0CF102A7   00000004    8        30\t75\tE0\t2E\t80\tFF\tFF\tFD\r\n      2823  0CF101A7   00000004    8        68\t00\t97\tCC\t00\t16\t39\tA7\r\n      2822  1FFFFFFF   00000004    8        00\t00\tFF\tFF\tFF\tFF\tFF\tFF\r\n      2812  1FFFFFFF   00000004    8        00\t00\tFF\tFF\tFF\tFF\tFF\tFF\r\n      2803  0CF102A7   00000004    8        30\t75\tE0\t2E\t80\tFF\tFF\tFD\r\n      2844  0CF103A7   00000004    8        17\t1F\t08\t60\tB1\t1F\t08\t54\r\n      2844  0CF102A7   00000004    8        30\t75\tE0\t2E\t80\tFF\tFF\tFD\r\n      2843  0C3C4D4A   00000004    8        BE\tFF\tFF\t7F\t18\tFF\tFF\t54\r\n      2843  0CF101A7   00000004    8        68\t00\t97\tCC\t00\t16\t39\tA8\r\n      2842  18F120F0   00000004    8        2B\t75\t60\tB1\tB0\t01\tFF\tFF\r\n      2841  18F11FF0   00000004    8        FF\t3F\t90\t68\t88\t1B\t10\t4C\r\n      2832  1FFFFFFF   00000004    8        00\t00\tFF\tFF\tFF\tFF\tFF\tFF\r\n      2823  0CF102A7   00000004    8        30\t75\tE0\t2E\t80\tFF\tFF\tFD\r\n      2823  0CF101A7   00000004    8        68\t00\t97\tCC\t00\t16\t39\tA7\r\n      2822  1FFFFFFF   00000004    8        00\t00\tFF\tFF\tFF\tFF\tFF\tFF\r\n      2812  1FFFFFFF   00000004    8        00\t00\tFF\tFF\tFF\tFF\tFF\tFF\r\n      2845  0CF104A7   00000004    8        F0\t60\t22\tFC\tFF\tFF\tFF\t54\r\n      2844  0CF103A7   00000004    8        17\t1F\t08\t60\tB1\t1F\t08\t54\r\n      2844  0CF102A7   00000004    8        30\t75\tE0\t2E\t80\tFF\tFF\tFD\r\n      2843  0C3C4D4A   00000004    8        BE\tFF\tFF\t7F\t18\tFF\tFF\t54\r\n      2843  0CF101A7   00000004    8        68\t00\t97\tCC\t00\t16\t39\tA8\r\n      2842  18F120F0   00000004    8        2B\t75\t60\tB1\tB0\t01\tFF\tFF\r\n      2841  18F11FF0   00000004    8        FF\t3F\t90\t68\t88\t1B\t10\t4C\r\n      2832  1FFFFFFF   00000004    8        00\t00\tFF\tFF\tFF\tFF\tFF\tFF\r\n      2823  0CF102A7   00000004    8        30\t75\tE0\t2E\t80\tFF\tFF\tFD\r\n      2823  0CF101A7   00000004    8        68\t00\t97\tCC\t00\t16\t39\tA7\r\n      2822  1FFFFFFF   00000004    8        00\t00\tFF\tFF\tFF\tFF\tFF\tFF\r\n      2845  18F106A7   00000004    8        00\tF7\tFF\tFF\tFF\tFF\tFF\tA9\r\n      2845  0CF104A7   00000004    8        F0\t60\t22\tFC\tFF\tFF\tFF\t54\r\n      2844  0CF103A7   00000004    8        17\t1F\t08\t60\tB1\t1F\t08\t54\r\n      2844  0CF102A7   00000004    8        30\t75\tE0\t2E\t80\tFF\tFF\tFD\r\n      2843  0C3C4D4A   00000004    8        BE\tFF\tFF\t7F\t18\tFF\tFF\t54\r\n      2843  0CF101A7   00000004    8        68\t00\t97\tCC\t00\t16\t39\tA8\r\n      2842  18F120F0   00000004    8        2B\t75\t60\tB1\tB0\t01\tFF\tFF\r\n      2841  18F11FF0   00000004    8        FF\t3F\t90\t68\t88\t1B\t10\t4C\r\n      2832  1FFFFFFF   00000004    8        00\t00\tFF\tFF\tFF\tFF\tFF\tFF\r\n      2823  0CF102A7   00000004    8        30\t75\tE0\t2E\t80\tFF\tFF\tFD\r\n      2823  0CF101A7   00000004    8        68\t00\t97\tCC\t00\t16\t39\tA7\r\n      2846  18F121F0   00000004    8        09\t19\t00\t00\tFF\tFF\tB0\t01\r\n      2845  18F106A7   00000004    8        00\tF7\tFF\tFF\tFF\tFF\tFF\tA9\r\n      2845  0CF104A7   00000004    8        F0\t60\t22\tFC\tFF\tFF\tFF\t54\r\n      2844  0CF103A7   00000004    8        17\t1F\t08\t60\tB1\t1F\t08\t54\r\n      2844  0CF102A7   00000004    8        30\t75\tE0\t2E\t80\tFF\tFF\tFD\r\n      2843  0C3C4D4A   00000004    8        BE\tFF\tFF\t7F\t18\tFF\tFF\t54\r\n      2843  0CF101A7   00000004    8        68\t00\t97\tCC\t00\t16\t39\tA8\r\n      2842  18F120F0   00000004    8        2B\t75\t60\tB1\tB0\t01\tFF\tFF\r\n      2841  18F11FF0   00000004    8        FF\t3F\t90\t68\t88\t1B\t10\t4C\r\n      2832  1FFFFFFF   00000004    8        00\t00\tFF\tFF\tFF\tFF\tFF\tFF\r\n      2823  0CF102A7   00000004    8        30\t75\tE0\t2E\t80\tFF\tFF\tFD\r\n      2847  1FFFFFFF   00000004    8        00\t00\tFF\tFF\tFF\tFF\tFF\tFF\r\n      2846  18F121F0   00000004    8        09\t19\t00\t00\tFF\tFF\tB0\t01\r\n      2845  18F106A7   00000004    8        00\tF7\tFF\tFF\tFF\tFF\tFF\tA9\r\n      2845  0CF104A7   00000004    8        F0\t60\t22\tFC\tFF\tFF\tFF\t54\r\n      2844  0CF103A7   00000004    8        17\t1F\t08\t60\tB1\t1F\t08\t54\r\n      2844  0CF102A7   00000004    8        30\t75\tE0\t2E\t80\tFF\tFF\tFD\r\n      2843  0C3C4D4A   00000004    8        BE\tFF\tFF\t7F\t18\tFF\tFF\t54\r\n      2843  0CF101A7   00000004    8        68\t00\t97\tCC\t00\t16\t39\tA8\r\n      2842  18F120F0   00000004    8        2B\t75\t60\tB1\tB0\t01\tFF\tFF\r\n      2841  18F11FF0   00000004    8        FF\t3F\t90\t68\t88\t1B\t10\t4C\r\n      2832  1FFFFFFF   00000004    8        00\t00\tFF\tFF\tFF\tFF\tFF\tFF\r\n      2852  1FFFFFFF   00000004    8        00\t20\tFF\tFF\tFF\tFF\tFF\tFF\r\n      2847  1FFFFFFF   00000004    8        00\t00\tFF\tFF\tFF\tFF\tFF\tFF\r\n      2846  18F121F0   00000004    8        09\t19\t00\t00\tFF\tFF\tB0\t01\r\n      2845  18F106A7   00000004    8        00\tF7\tFF\tFF\tFF\tFF\tFF\tA9\r\n      2845  0CF104A7   00000004    8        F0\t60\t22\tFC\tFF\tFF\tFF\t54\r\n      2844  0CF103A7   00000004    8        17\t1F\t08\t60\tB1\t1F\t08\t54\r\n      2844  0CF102A7   00000004    8        30\t75\tE0\t2E\t80\tFF\tFF\tFD\r\n      2843  0C3C4D4A   00000004    8        BE\tFF\tFF\t7F\t18\tFF\tFF\t54\r\n      2843  0CF101A7   00000004    8        68\t00\t97\tCC\t00\t16\t39\tA8\r\n      2842  
